vi "GenerateFilepath.vi"(3 "Check for file?":bool=TRUE, 4 "File Information":T1={"Project"=0, "SubFolder"="Temp Dependence", "Filename (Meas. Description)"="200C", "Measurement number"=2} {"Project" items=["Proj_VaporTubes", "Proj_H2DT", "Proj_H2DT"]}, 5 "Instrument":string="Control") -> (0 "File Action":i32=2, 1 "File Information Out":T1={"Project"=1, "SubFolder"="Temp Dependence", "Filename (Meas. Description)"="200C", "Measurement number"=0} {"Project" items=["Proj_VaporTubes", "Proj_H2DT", "Proj_H2DT"]}, 2 "File Path Out":path=path "D:/Data/2018-06-15/Proj_1/Temp Dependence/Control_200C.tdms")   [LabVIEW 2018]
uses:
  <vilib>/Utility/file.llb/Read Delimited Spreadsheet (string).vi
panel:
  in  "Path":path=path "E:/ProjectIndex.csv"
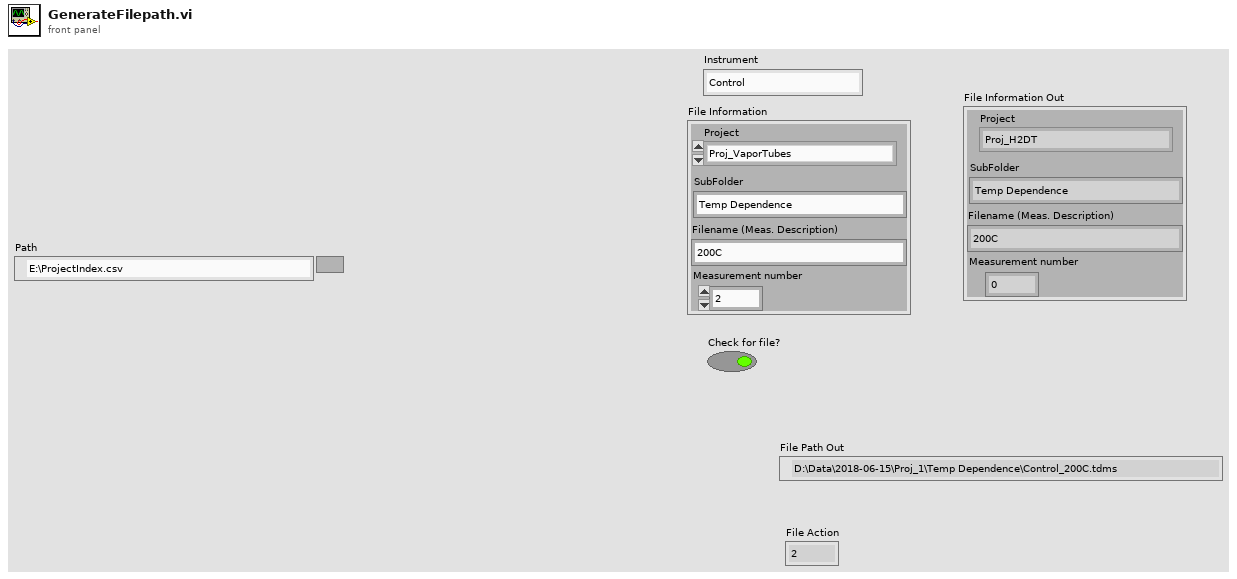
[diagram p1: front panel]
types:
  T1 = cluster{"Project":u16, "SubFolder":string, "Filename (Meas. Description)":string, "Measurement number":i32}
  T2 = enum16{"open", "open or create", "create or replace", "create", "open (read-only)"}
  T3 = cluster{"Project":u16, "SubFolder 2":string, "Meas. Description 2":string, "Measurement number 2":i32}
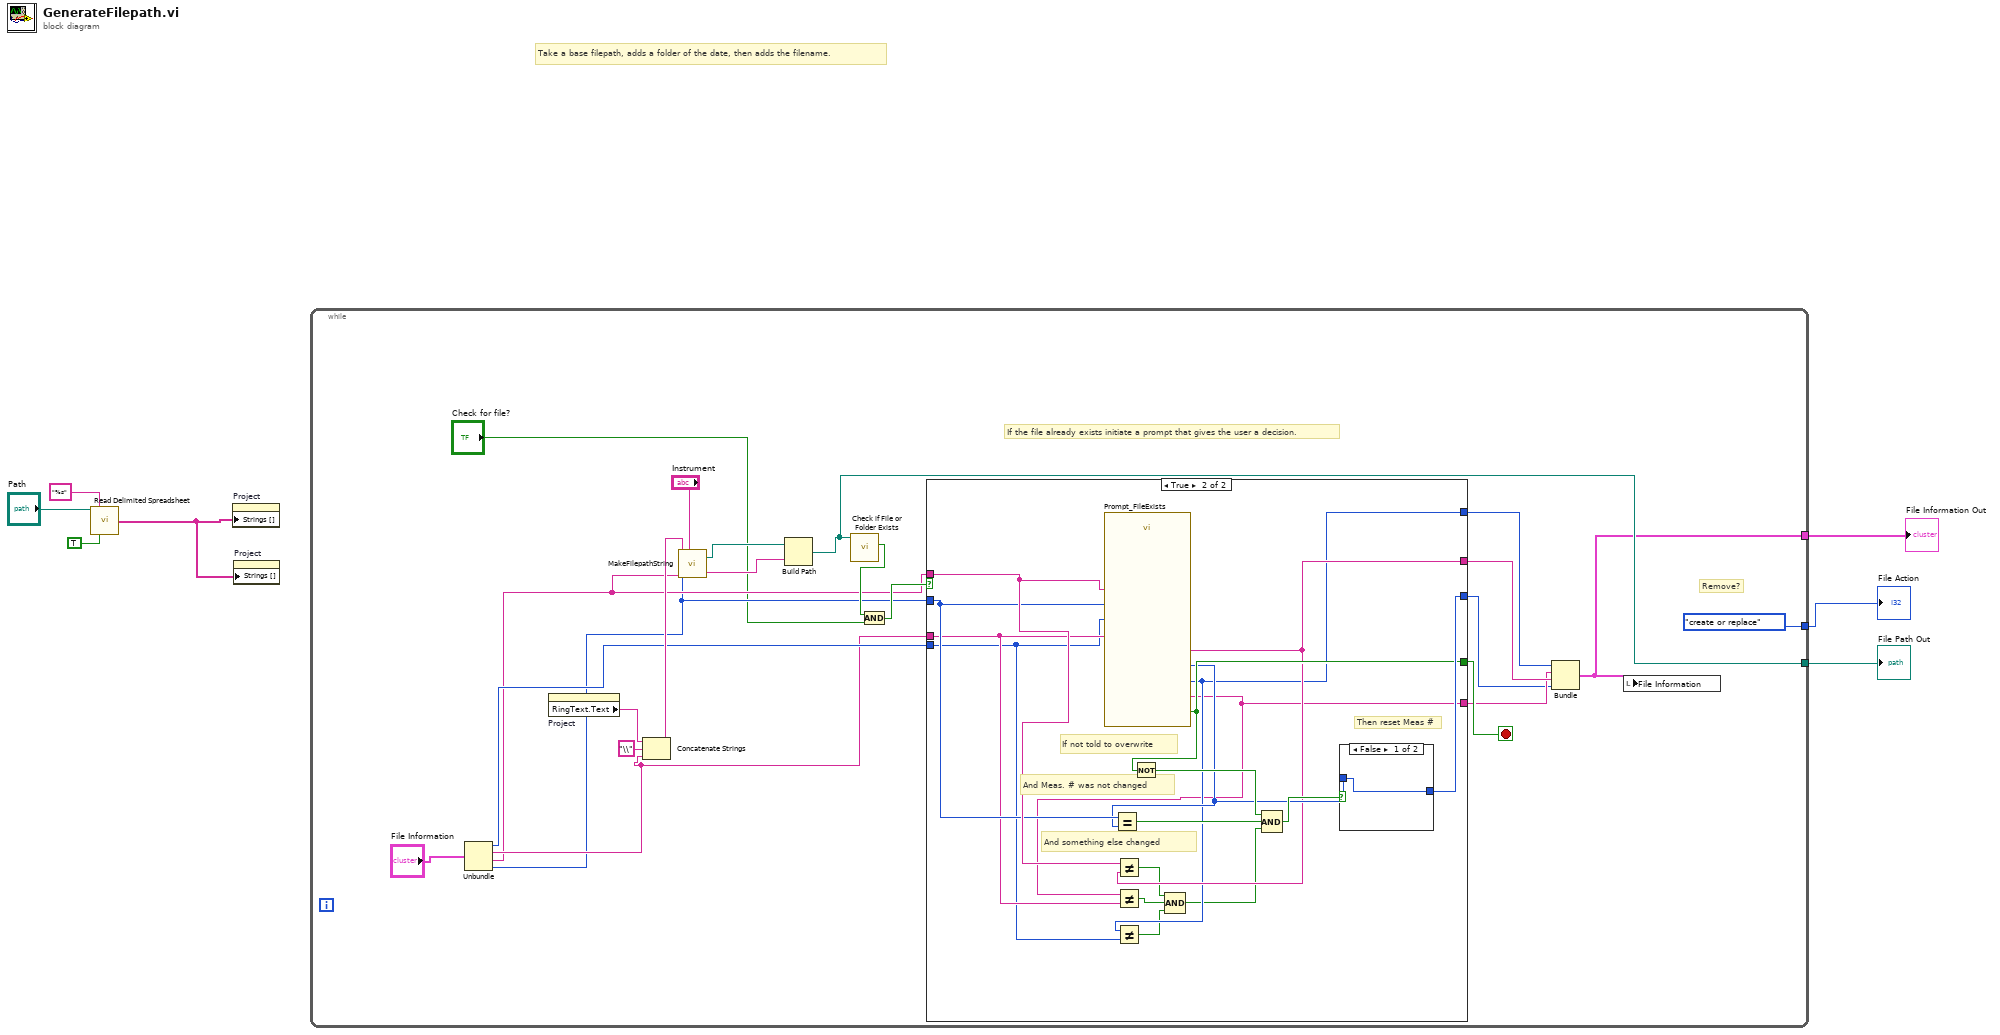
[diagram p0: block diagram]
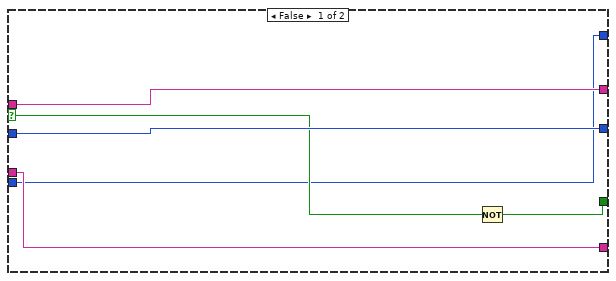
[diagram p2: hidden frame]
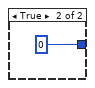
[diagram p3: hidden frame]
diagram:
  # "Take a base filepath, adds a folder of the date, then adds the filename."
  n1 = call-poly <vilib>:"Read Delimited Spreadsheet.vi"("file path (dialog if empty)"="Path", "format (%s)"="%s", "transpose? (F)"=TRUE) -> ("first row"=w1:string[])  [unwired: 7 in, 5 out]
  n2 = property on="Project" class="Ring (strict)"("Strings []"=w1) -> ()  [unwired: 2 in, 2 out]
  n3 = property on="Project" class="Ring (strict)"("Strings []"=w1) -> ()  [unwired: 2 in, 2 out]
  n4 = while {
    tunnel: [T2."create or replace" ("operation (0:open)")] -> w7
    tunnel: [w24] -> w6
    tunnel: [w10] -> w5
    stop <- w25 stop-if-true
    # "Remove?"
    # "If the file already exists initiate a prompt that gives the user a decision."
    n5 = Unbundle("File Information") -> ("Project"=w18:u16, "SubFolder"=w17:string, "Filename (Meas. Description)"=w16:string, "Measurement number"=w15:i32)
    n6 = property on="Project" class="Ring (strict)"() -> ("RingText.Text"=w8:string)  [unwired: 2 in, 2 out]
    n7 = Concatenate Strings(w8, "\\" ("string"), w17) -> (w22:string)
    n8 = call "MakeFilepathString.vi"("Project"=w22, "Measurement number"=w15, "Extra"=w16, "Instrument"="Instrument") -> ("Folder"=w27:path, "Filename"=w26:string)  [unwired: 1 in]
    n9 = Build Path(base path=w27, name or relative path=w26) -> (appended path=w24:path)
    n10 = call <vilib>:"Check if File or Folder Exists.vi"("path"=w24) -> ("file or folder exists?"=w20:bool)  [unwired: 8 in, 2 out]
    n11 = And(x=w20, y="Check for file?") -> (x .and. y?=w21:bool)
    n12 = case shown="True" w21 {
      selector: w21 -> [w33 _]
      tunnel: w15 -> [w35 w47]
      tunnel: w16 -> [w34 w48]
      tunnel: [w30 w40] -> w12
      tunnel: [w34 w44] -> w14
      tunnel: [w35 w52] -> w11
      tunnel: [w32 w46] -> w25
      tunnel: w18 -> [w30 w39]
      tunnel: w17 -> [w31 w43]
      tunnel: [w31 w36] -> w13
      frame False {
        n13 = Not(x=w33) -> (.not. x?=w32:bool)
      }
      frame True {
        # "Then reset Meas #"
        # "And something else changed"
        # "And Meas. # was not changed"
        # "If not told to overwrite"
        n14 = call "Prompt_FileExists.vi"("Project"=w39, "SubFolder"=w43, "Meas. Description"=w48, "Measurement number"=w47) -> ("Measurement number 2"=w45:i32, "Project 2"=w40:enum16{"H2TC", "VAPOR1"}, "SubFolder 2"=w36:string, "Meas. Description 2"=w44:string, "Overwrite"=w46:bool)
        n15 = Equal?(x=w47, y=w45) -> (x = y?=w50:bool)
        n16 = Not Equal?(x=w48, y=w44) -> (x != y?=w42:bool)
        n17 = Not Equal?(x=w36, y=w43) -> (x != y?=w41:bool)
        n18 = Not Equal?(x=w40, y=w39) -> (x != y?=w38:bool)
        n19 = Not(x=w46) -> (.not. x?=w51:bool)
        n20 = Compound Arithmetic op=AND(w42, w41, w38) -> (w37:bool)
        n21 = Compound Arithmetic op=AND(w51, w50, w37) -> (w49:bool)
        n22 = case shown="False" w49 {
          tunnel: w45 -> [w53 _]
          tunnel: [w53 0] -> w52
          frame False {
          }
          frame True {
          }
        }
      }
    }
    n23 = Bundle("Project"=w12, "SubFolder 2"=w13, "Meas. Description 2"=w14, "Measurement number 2"=w11) -> (w10:T3)  [unwired: 1 in]
    n24 = local write "File Information"(w10) -> ()
  }
  "File Action" <- w7
  "File Path Out" <- w6
  "File Information Out" <- w5
